vi "cake size.vi"(7 "shape":enum16{"round", "rectangle", "triangle"}(ring), 8 "theta":dbl format="%#_13g", 9 "b":dbl format="%#_13g", 10 "a":dbl format="%#_13g", 11 "r":dbl format="%#_13g") -> (2 "size":dbl)   [LabVIEW 2023]
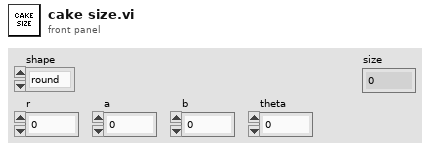
[diagram p1: front panel]
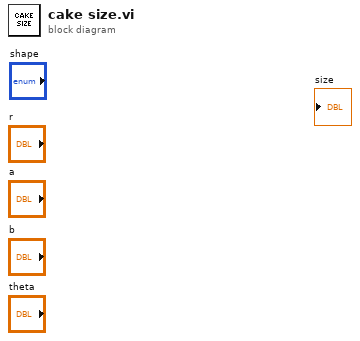
[diagram p0: block diagram]
diagram:
